vi "Teleop.vi"() -> ()   [LabVIEW 2015]
doc: "This VI is called for each TeleOp packet received from the DS where the robot is not disabled. It is often used to read from the joysticks and update I/O or to update setpoints for timed control loops. It should complete and return within 20 milliseconds or it may miss DS packets."
uses:
  <vilib>/Rock Robotics/WPI/DriverStation/WPI_DriverStationDerivedRobotMode.ctl
  <vilib>/Rock Robotics/WPI/DriverStation/WPI_DriverStationMatch Info.ctl
  <vilib>/Rock Robotics/Network Tables/NT Read Boolean.vi
  <vilib>/Rock Robotics/Network Tables/NT Read Number.vi
  <vilib>/Rock Robotics/Network Tables/SD Read Boolean.vi
  <vilib>/Rock Robotics/Network Tables/SD Read Number.vi
  <vilib>/Rock Robotics/WPI/Utilities/WPI_GetSetVariantRefNum.vi
  <vilib>/Rock Robotics/Network Tables/SD Write Number.vi
panel:
  out "final_test":dbl
  out "test":dbl
  out "Sample Slider 1":dbl(slide) scale=0.0..5.0
  out "Sample Boolean 3":bool
  out "Sample Boolean 2":bool
  in  "Match Info":T1={"Autonomous Elapsed Seconds"=0.0, "TeleOp Elapsed Seconds"=0.0, "Disabled Elapsed Seconds"=0.0, "Visited Autonomous"=FALSE, "Visited TeleOp"=FALSE, "Visited Disabled"=FALSE, "Autonomous Settings"={"Autonomous Style"=enum."Independent", "VI Refnum"=refnum}}
  in  "Call Context":T2
  out "Sample Slider 0":dbl(slide) scale=0.0..5.0
  out "Sample Boolean 1":bool
  out "Sample Boolean 0":bool
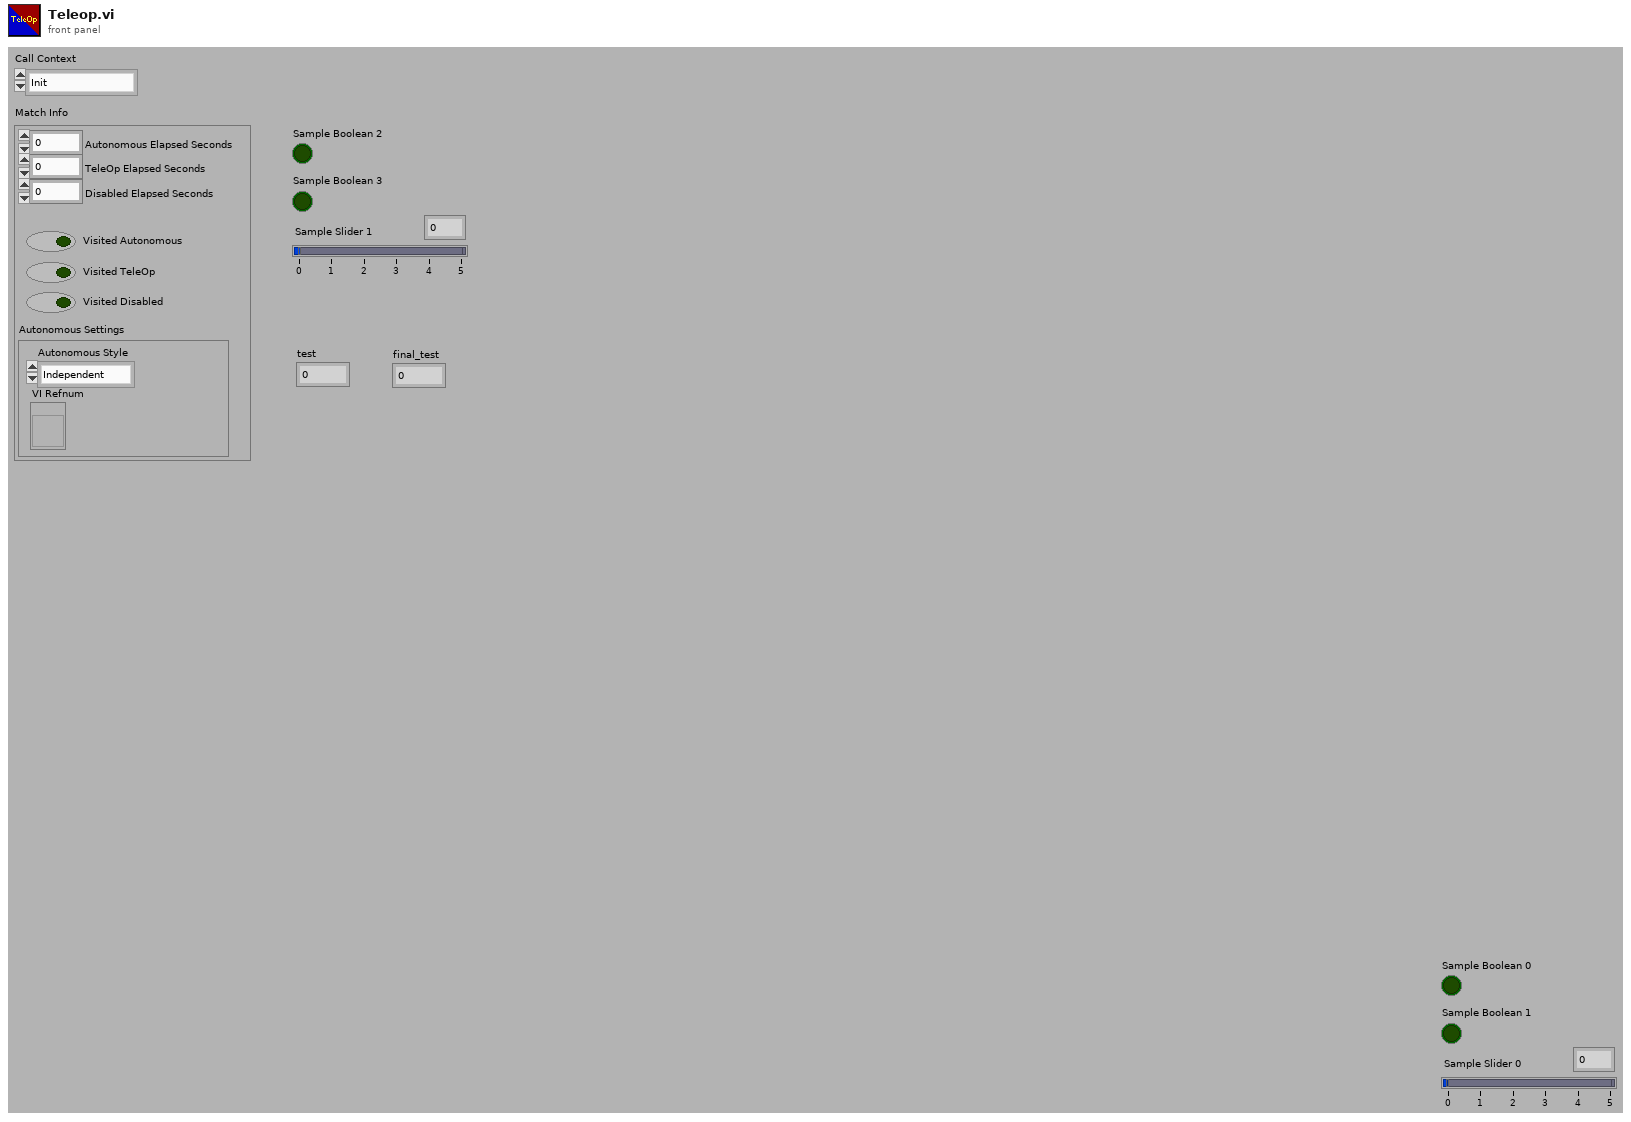
[diagram p1: front panel]
types:
  T1 = typedef "WPI_DriverStationMatch Info.ctl" = cluster{"Autonomous Elapsed Seconds":dbl, "TeleOp Elapsed Seconds":dbl, "Disabled Elapsed Seconds":dbl, "Visited Autonomous":bool, "Visited TeleOp":bool, "Visited Disabled":bool, "Autonomous Settings":cluster{"Autonomous Style":enum16{"Iterative", "Independent"}, "VI Refnum":refnum<vi>}}
  T2 = typedef "WPI_DriverStationDerivedRobotMode.ctl" = enum16{"Init", "Execute", "Stop"}
  T3 = typedef "WPI_JoystickDevRef.ctl" = cluster{"Device":T4}
  T4 = typedef "WPI_JoystickDeviceEnum.ctl" = enum16{"USB 0", "USB 1", "USB 2", "USB 3", "USB 4", "USB 5"}
  T5 = cluster{"Axes[0]":dbl, "Axes[1]":dbl, "Axes[2]":dbl, "Axes[3]":dbl, "Axes[4]":dbl, "Axes[5]":dbl, "Axes[6]":dbl, "Axes[7]":dbl, "Axes[8]":dbl}
  T6 = typedef "WPI_EncoderDevRef.ctl" = cluster{"DevStatus":errorcluster, "EncoderIndex":T7, "CounterIndex":T8, "DistancePerCount":dbl, "Decoding Type":T9}
  T7 = typedef "FPGA_EncoderIdx.ctl" = enum8{"Enc 0", "Enc 1", "Enc 2", "Enc 3", "Enc 4", "Enc 5", "Enc 6", "Enc 7", "Invalid"}
  T8 = typedef "FPGA_CounterCtrSystemIndex.ctl" = enum8{"Ctr 0", "Ctr 1", "Ctr 2", "Ctr 3", "Ctr 4", "Ctr 5", "Ctr 6", "Ctr 7", "Invalid"}
  T9 = typedef "WPI_EncoderType.ctl" = enum16{"1x", "2x", "4x"}
  T10 = typedef "WPI_RobotDriveDevRef.ctl" = cluster{"DevStatus":errorcluster, "Motors[]":T11[], "Square Inputs":bool, "Max Output":dbl}
  T11 = typedef "WPI_MotorControlDeviceRef.ctl" = cluster{"DeviceStatus":errorcluster, "Type":T12, "PWM":cluster{"PWM Channel":T13, "DeadBand":T14}, "CAN":cluster{"Device Number":u8, "Control Mode":T15, "Semaphore":T16, "Max Vout":dbl, "TalonSRX Control Mode":T17}, "Invert":bool}
  T12 = typedef "WPI_MotorControlType.ctl" = enum16{"PWM", "CAN", "CANTalonSRX"}
  T13 = typedef "FPGA_DIOPWMChannel.ctl" = enum8{"PWM 0", "PWM 1", "PWM 2", "PWM 3", "PWM 4", "PWM 5", "PWM 6", "PWM 7", "PWM 8", "PWM 9", "PWM MXP 0", "PWM MXP 1", "PWM MXP 2", "PWM MXP 3", "PWM MXP 4", "PWM MXP 5", "PWM MXP 6", "PWM MXP 7", "PWM MXP 8", "PWM MXP 9", "Invalid"}
  T14 = typedef "WPI_PWMDeadband.ctl" = cluster{"Name":string, "maxPositivePwm":i32, "minPositivePwm":i32, "centerPwm":i32, "maxNegativePwm":i32, "minNegativePwm":i32, "angularRange":u16}
  T15 = typedef "WPI_CANJaguar_ControlMode.ctl" = enum8{"Percent VBus", "Current", "Speed", "Position", "Voltage"}
  T16 = typedef "Semaphore RefNum" = refnum<k1>
  T17 = typedef "WPI_CANTalonSRX_APIControlMode.ctl" = enum8{"Percent VBus", "Speed", "Position", "Slave", "Unchanged / Invalid", "Voltage Compensation", "Current", "Motion Profile"}
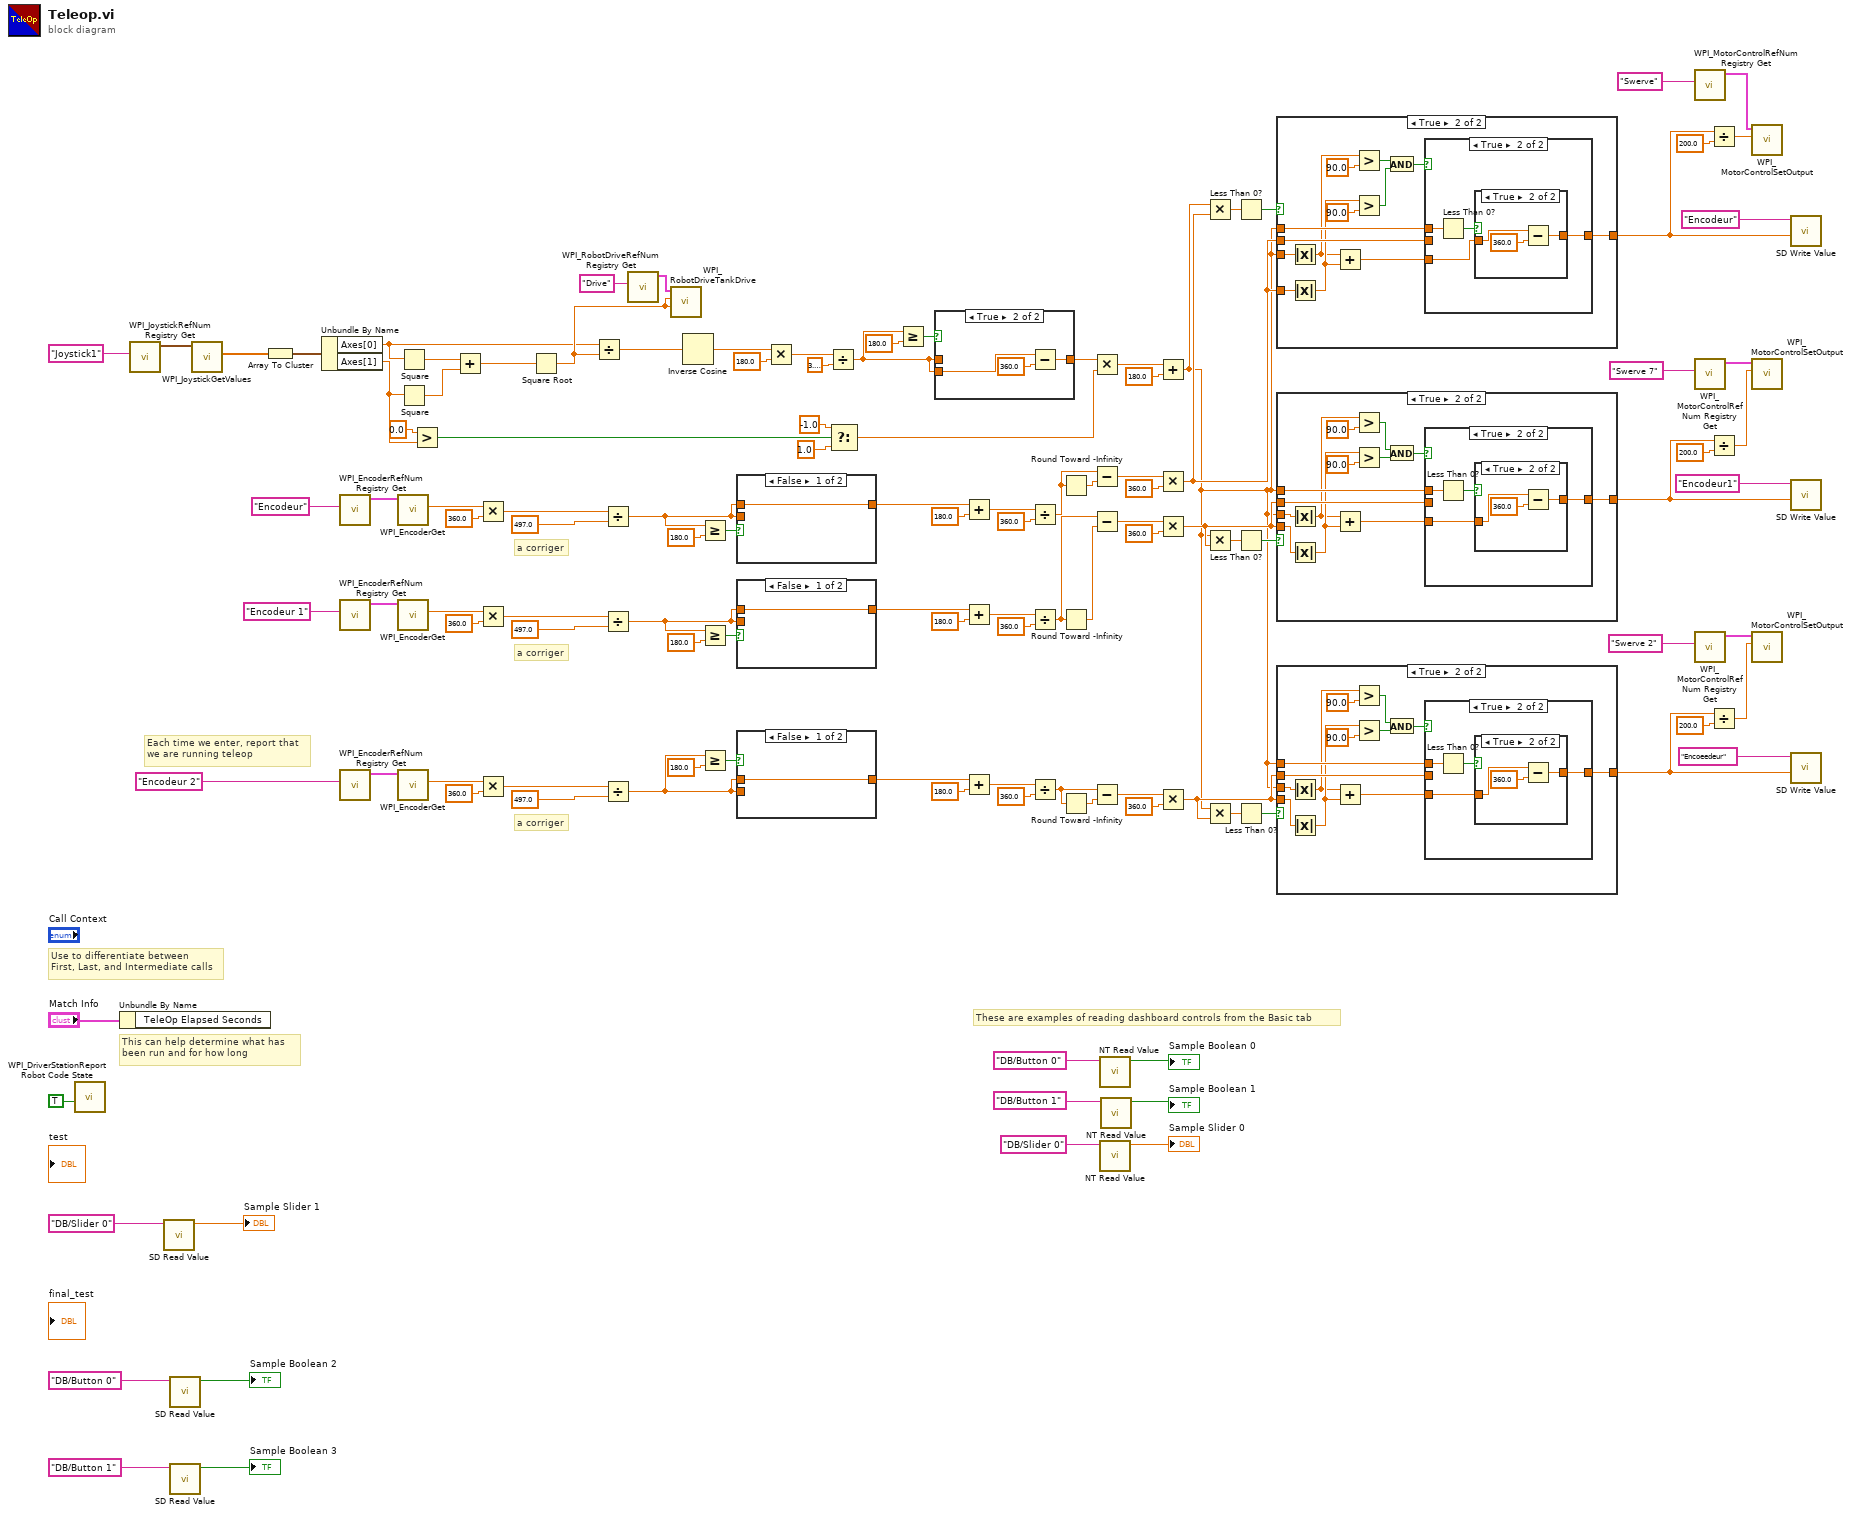
[diagram p0: block diagram]
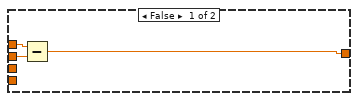
[diagram p2: hidden frame]
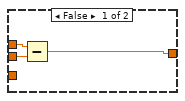
[diagram p3: hidden frame]
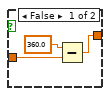
[diagram p4: hidden frame]
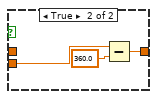
[diagram p5: hidden frame]
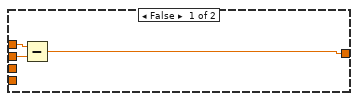
[diagram p6: hidden frame]
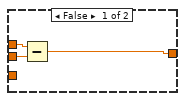
[diagram p7: hidden frame]
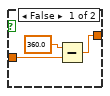
[diagram p8: hidden frame]
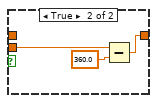
[diagram p9: hidden frame]
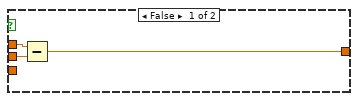
[diagram p10: hidden frame]
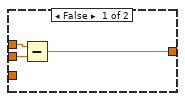
[diagram p11: hidden frame]
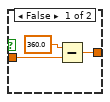
[diagram p12: hidden frame]
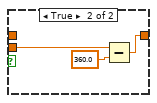
[diagram p13: hidden frame]
diagram:
  # "a corriger"
  # "a corriger"
  # "a corriger"
  # "Each time we enter, report that\nwe are running teleop"
  # "Use to differentiate between\nFirst, Last, and Intermediate calls"
  # "This can help determine what has\nbeen run and for how long"
  # "These are examples of reading dashboard controls from the Basic tab"
  n1 = call <vilib>:"WPI_DriverStationReport Robot Code State.vi"("TeleOp"=TRUE ("Autonomous")) -> ()  [unwired: 10 in, 1 out]
  n2 = Unbundle By Name("Match Info") -> ()  [unwired: 1 out]
  n3 = call <vilib>:"WPI_JoystickRefNum Registry Get.vi"("refnum name"="Joystick1") -> ("JoystickDevRef"=w107:T3)  [unwired: 9 in, 1 out]
  n4 = call-poly <vilib>:"SD Read Value.vi"("Name"="DB/Slider 0" ("refnum name")) -> ("Numeric"=→"Sample Slider 1":dbl)  [unwired: 8 in, 2 out]
  n5 = call-poly <vilib>:"SD Read Value.vi"("Name"="DB/Button 0" ("refnum name")) -> ("Boolean"=→"Sample Boolean 2":bool)  [unwired: 8 in, 2 out]
  n6 = call-poly <vilib>:"SD Read Value.vi"("Name"="DB/Button 1" ("refnum name")) -> ("Boolean"=→"Sample Boolean 3":bool)  [unwired: 8 in, 2 out]
  n7 = call <vilib>:"WPI_JoystickGetValues.vi"("JoystickDevRef"=w107) -> ("Axes"=w105:dbl[])  [unwired: 6 in, 4 out]
  n8 = Array To Cluster(array=w105) -> (cluster=w104:T5)
  n9 = Unbundle By Name(w104) -> ("Axes[0]"=w56:dbl, "Axes[1]"=w55:dbl)
  n10 = call <vilib>:"WPI_EncoderRefNum Registry Get.vi"("refnum name"="Encodeur") -> ("EncoderDevRef"=w100:T6)  [unwired: 9 in, 1 out]
  n11 = call <vilib>:"WPI_EncoderRefNum Registry Get.vi"("refnum name"="Encodeur 1") -> ("EncoderDevRef"=w52:T6)  [unwired: 9 in, 1 out]
  n12 = call <vilib>:"WPI_EncoderRefNum Registry Get.vi"("refnum name"="Encodeur 2") -> ("EncoderDevRef"=w24:T6)  [unwired: 9 in, 1 out]
  n13 = call <vilib>:"WPI_EncoderGet.vi"("EncoderDevRef"=w100) -> ("Distance"=w54:dbl)  [unwired: 5 in, 5 out]
  n14 = call <vilib>:"WPI_EncoderGet.vi"("EncoderDevRef"=w52) -> ("Distance"=w37:dbl)  [unwired: 5 in, 5 out]
  n15 = call <vilib>:"WPI_EncoderGet.vi"("EncoderDevRef"=w24) -> ("Distance"=w2:dbl)  [unwired: 5 in, 5 out]
  n16 = Square(x=w56) -> (x^2=w98:dbl)
  n17 = Square(x=w55) -> (x^2=w99:dbl)
  n18 = Greater?(x=0.0, y=w55) -> (0:w83:bool)
  n19 = Add(x=w98, y=w99) -> (x+y=w97:dbl)
  n20 = Multiply(x=w54, y=360.0) -> (x*y=w91:dbl)
  n21 = Multiply(x=w37, y=360.0) -> (x*y=w50:dbl)
  n22 = Multiply(x=w2, y=360.0) -> (x*y=w22:dbl)
  n23 = Square Root(x=w97) -> (sqrt(x)=w62:dbl)
  n24 = Divide(x=w56, y=w62) -> (x/y=w96:dbl)
  n25 = Divide(x=w91, y=497.0) -> (x/y=w75:dbl)
  n26 = Divide(x=w50, y=497.0) -> (x/y=w46:dbl)
  n27 = Divide(x=w22, y=497.0) -> (x/y=w16:dbl)
  n28 = call <vilib>:"WPI_RobotDriveRefNum Registry Get.vi"("refnum name"="Drive") -> ("RobotDriveDevRef"=w63:T10)  [unwired: 9 in, 1 out]
  n29 = call <vilib>:"WPI_RobotDriveTankDrive.vi"("Right axis value"=w62, "Left axis value"=w62, "RobotDriveDevRef"=w63) -> ()  [unwired: 6 in, 3 out]
  n30 = Inverse Cosine(1:w96) -> (0:w84:dbl)
  n31 = Greater Or Equal?(x=w75, y=180.0) -> (x >= y?=w76:bool)
  n32 = Greater Or Equal?(x=w46, y=180.0) -> (x >= y?=w47:bool)
  n33 = Greater Or Equal?(x=w16, y=180.0) -> (x >= y?=w17:bool)
  n34 = case shown="False" w76 {
    tunnel: w75 -> [_ w124]
    tunnel: [w122 w123] -> w72
    tunnel: w75 -> [w122 _]
    frame False {
    }
    frame True {
      n35 = Subtract(x=w124, y=360.0) -> (x-y=w123:dbl)
    }
  }
  n36 = case shown="False" w47 {
    tunnel: w46 -> [_ w128]
    tunnel: [w126 w127] -> w45
    tunnel: w46 -> [w126 _]
    frame False {
    }
    frame True {
      n37 = Subtract(x=w128, y=360.0) -> (x-y=w127:dbl)
    }
  }
  n38 = case shown="False" w17 {
    tunnel: w16 -> [_ w132]
    tunnel: [w130 w131] -> w15
    tunnel: w16 -> [w130 _]
    frame False {
    }
    frame True {
      n39 = Subtract(x=w132, y=360.0) -> (x-y=w131:dbl)
    }
  }
  n40 = Multiply(x=w84, y=180.0) -> (x*y=w94:dbl)
  n41 = Divide(x=w94, y=3.141592653589793) -> (x/y=w78:dbl)
  n42 = Select(t=-1.0, s=w83, f=1.0) -> (s? t:f=w79:dbl)
  n43 = Greater Or Equal?(x=w78, y=180.0) -> (x >= y?=w86:bool)
  n44 = case shown="True" w86 {
    tunnel: w78 -> [_ w136]
    tunnel: [w134 w135] -> w80
    tunnel: w78 -> [w134 _]
    frame False {
    }
    frame True {
      n45 = Subtract(x=w136, y=360.0) -> (x-y=w135:dbl)
    }
  }
  n46 = Add(x=w72, y=180.0) -> (x+y=w70:dbl)
  n47 = Add(x=w45, y=180.0) -> (x+y=w43:dbl)
  n48 = Add(x=w15, y=180.0) -> (x+y=w13:dbl)
  n49 = Divide(x=w70, y=360.0) -> (x/y=w67:dbl)
  n50 = Divide(x=w43, y=360.0) -> (x/y=w40:dbl)
  n51 = Divide(x=w13, y=360.0) -> (x/y=w10:dbl)
  n52 = Round Toward -Infinity(1:w67) -> (0:w68:dbl)
  n53 = Round Toward -Infinity(1:w40) -> (0:w41:dbl)
  n54 = Round Toward -Infinity(1:w10) -> (0:w11:dbl)
  n55 = Multiply(x=w80, y=w79) -> (x*y=w74:dbl)
  n56 = Subtract(x=w67, y=w68) -> (x-y=w65:dbl)
  n57 = Subtract(x=w40, y=w41) -> (x-y=w38:dbl)
  n58 = Subtract(x=w10, y=w11) -> (x-y=w8:dbl)
  n59 = call-poly <vilib>:"NT Read Value.vi"("Name"="DB/Button 0" ("refnum name")) -> ("Boolean"=→"Sample Boolean 0":bool)  [unwired: 9 in, 1 out]
  n60 = call-poly <vilib>:"NT Read Value.vi"("Name"="DB/Slider 0" ("refnum name")) -> ("Numeric"=→"Sample Slider 0":dbl)  [unwired: 9 in, 1 out]
  n61 = call-poly <vilib>:"NT Read Value.vi"("Name"="DB/Button 1" ("refnum name")) -> ("Boolean"=→"Sample Boolean 1":bool)  [unwired: 9 in, 1 out]
  n62 = Add(x=w74, y=180.0) -> (x+y=w1:dbl)
  n63 = Multiply(x=w65, y=360.0) -> (x*y=w59:dbl)
  n64 = Multiply(x=w38, y=360.0) -> (x*y=w28:dbl)
  n65 = Multiply(x=w8, y=360.0) -> (x*y=w5:dbl)
  n66 = Multiply(x=w1, y=w59) -> (x*y=w61:dbl)
  n67 = Multiply(x=w1, y=w28) -> (x*y=w32:dbl)
  n68 = Multiply(x=w1, y=w5) -> (x*y=w7:dbl)
  n69 = Less Than 0?(x=w61) -> (x < 0?=w60:bool)
  n70 = Less Than 0?(x=w32) -> (x < 0?=w31:bool)
  n71 = Less Than 0?(x=w7) -> (x < 0?=w6:bool)
  n72 = case shown="True" w60 {
    tunnel: [w140 w153] -> w58
    tunnel: w1 -> [w139 w152]
    tunnel: w59 -> [w138 w151]
    tunnel: w1 -> [_ w145]
    tunnel: w59 -> [_ w144]
    frame False {
      n73 = Subtract(x=w139, y=w138) -> (x-y=w140:dbl)
    }
    frame True {
      n74 = Absolute Value(x=w145) -> (abs(x)=w142:dbl)
      n75 = Absolute Value(x=w144) -> (abs(x)=w143:dbl)
      n76 = Add(x=w142, y=w143) -> (x+y=w141:dbl)
      n77 = Greater?(x=w142, y=90.0) -> (0:w147:bool)
      n78 = Greater?(x=w143, y=90.0) -> (0:w146:bool)
      n79 = And(x=w147, y=w146) -> (x .and. y?=w150:bool)
      n80 = case shown="True" w150 {
        tunnel: [w154 w159] -> w153
        tunnel: w152 -> [w156 w158]
        tunnel: w151 -> [w155 _]
        tunnel: w141 -> [_ w157]
        frame False {
          n81 = Subtract(x=w156, y=w155) -> (x-y=w154:dbl)
        }
        frame True {
          n82 = Less Than 0?(x=w158) -> (x < 0?=w160:bool)
          n83 = case shown="True" w160 {
            tunnel: [w163 w166] -> w159
            tunnel: w157 -> [w161 w164]
            frame False {
              n84 = Subtract(x=360.0 ("y"), y=w161) -> (x-y=w163:dbl)
            }
            frame True {
              n85 = Subtract(x=w164, y=360.0 ("x")) -> (x-y=w166:dbl)
            }
          }
        }
      }
    }
  }
  n86 = case shown="True" w31 {
    tunnel: [w169 w182] -> w30
    tunnel: w1 -> [w168 w181]
    tunnel: w28 -> [w167 w180]
    tunnel: w1 -> [_ w174]
    tunnel: w28 -> [_ w173]
    frame False {
      n87 = Subtract(x=w168, y=w167) -> (x-y=w169:dbl)
    }
    frame True {
      n88 = Absolute Value(x=w174) -> (abs(x)=w171:dbl)
      n89 = Absolute Value(x=w173) -> (abs(x)=w172:dbl)
      n90 = Add(x=w171, y=w172) -> (x+y=w170:dbl)
      n91 = Greater?(x=w171, y=90.0) -> (0:w176:bool)
      n92 = Greater?(x=w172, y=90.0) -> (0:w175:bool)
      n93 = And(x=w176, y=w175) -> (x .and. y?=w179:bool)
      n94 = case shown="True" w179 {
        tunnel: [w183 w188] -> w182
        tunnel: w181 -> [w185 w187]
        tunnel: w180 -> [w184 _]
        tunnel: w170 -> [_ w186]
        frame False {
          n95 = Subtract(x=w185, y=w184) -> (x-y=w183:dbl)
        }
        frame True {
          n96 = Less Than 0?(x=w187) -> (x < 0?=w189:bool)
          n97 = case shown="True" w189 {
            tunnel: [w192 w195] -> w188
            tunnel: w186 -> [w190 w193]
            frame False {
              n98 = Subtract(x=360.0 ("y"), y=w190) -> (x-y=w192:dbl)
            }
            frame True {
              n99 = Subtract(x=w193, y=360.0 ("x")) -> (x-y=w195:dbl)
            }
          }
        }
      }
    }
  }
  n100 = case shown="True" w6 {
    tunnel: [w198 w211] -> w4
    tunnel: w1 -> [w197 w210]
    tunnel: w5 -> [w196 w209]
    tunnel: w1 -> [_ w203]
    tunnel: w5 -> [_ w202]
    frame False {
      n101 = Subtract(x=w197, y=w196) -> (x-y=w198:dbl)
    }
    frame True {
      n102 = Absolute Value(x=w203) -> (abs(x)=w200:dbl)
      n103 = Absolute Value(x=w202) -> (abs(x)=w201:dbl)
      n104 = Add(x=w200, y=w201) -> (x+y=w199:dbl)
      n105 = Greater?(x=w200, y=90.0) -> (0:w205:bool)
      n106 = Greater?(x=w201, y=90.0) -> (0:w204:bool)
      n107 = And(x=w205, y=w204) -> (x .and. y?=w208:bool)
      n108 = case shown="True" w208 {
        tunnel: [w212 w217] -> w211
        tunnel: w210 -> [w214 w216]
        tunnel: w209 -> [w213 _]
        tunnel: w199 -> [_ w215]
        frame False {
          n109 = Subtract(x=w214, y=w213) -> (x-y=w212:dbl)
        }
        frame True {
          n110 = Less Than 0?(x=w216) -> (x < 0?=w218:bool)
          n111 = case shown="True" w218 {
            tunnel: [w221 w224] -> w217
            tunnel: w215 -> [w219 w222]
            frame False {
              n112 = Subtract(x=360.0 ("y"), y=w219) -> (x-y=w221:dbl)
            }
            frame True {
              n113 = Subtract(x=w222, y=360.0 ("x")) -> (x-y=w224:dbl)
            }
          }
        }
      }
    }
  }
  n114 = call <vilib>:"WPI_MotorControlRefNum Registry Get.vi"("refnum name"="Swerve") -> ("MotorControlDevRef"=w102:T11)  [unwired: 9 in, 1 out]
  n115 = call <vilib>:"WPI_MotorControlRefNum Registry Get.vi"("refnum name"="Swerve 7") -> ("MotorControlDevRef"=w35:T11)  [unwired: 9 in, 1 out]
  n116 = call <vilib>:"WPI_MotorControlRefNum Registry Get.vi"("refnum name"="Swerve 2") -> ("MotorControlDevRef"=w26:T11)  [unwired: 9 in, 1 out]
  n117 = Divide(x=w58, y=200.0) -> (x/y=w88:dbl)
  n118 = Divide(x=w30, y=200.0) -> (x/y=w33:dbl)
  n119 = Divide(x=w4, y=200.0) -> (x/y=w19:dbl)
  n120 = call <vilib>:"WPI_MotorControlSetOutput.vi"("Output"=w88, "MotorControlDevRef"=w102) -> ()  [unwired: 7 in, 3 out]
  n121 = call <vilib>:"WPI_MotorControlSetOutput.vi"("Output"=w33, "MotorControlDevRef"=w35) -> ()  [unwired: 7 in, 3 out]
  n122 = call <vilib>:"WPI_MotorControlSetOutput.vi"("Output"=w19, "MotorControlDevRef"=w26) -> ()  [unwired: 7 in, 3 out]
  n123 = call-poly <vilib>:"SD Write Value.vi"("Numeric"=w58, "Name"="Encodeur") -> ()  [unwired: 8 in, 2 out]
  n124 = call-poly <vilib>:"SD Write Value.vi"("Numeric"=w30, "Name"="Encodeur1") -> ()  [unwired: 8 in, 2 out]
  n125 = call-poly <vilib>:"SD Write Value.vi"("Numeric"=w4, "Name"="Encoeedeur") -> ()  [unwired: 8 in, 2 out]
